vi "Save_to_Project.vi"(8 "error in (no error)":errorcluster, 9 "index in":string, 10 "buildObject":T2, 11 "IB_SoftDependency in":refnum<class "IB_SoftDependency.lvclass">) -> (0 "error out":errorcluster, 1 "index out":string, 2 "buildObject out":T2, 3 "IB_SoftDependency out":refnum<class "IB_SoftDependency.lvclass">)   [LabVIEW 2020, in "IB_SoftDependency.lvclass"]
uses:
  <vilib>/AppBuilder/IB_Classes/SoftDependency/IB_SoftDependency.lvclass
  <vilib>/AppBuilder/IB_Classes/SoftDependency/IB_SoftDependency.lvclass/IB_SoftDependency.ctl
  <vilib>/AppBuilder/IB_RW_Project/IB_RW_Project_PropBag_Action.ctl
  <resource>/Framework/Providers/API/ItemRef.ctl
  <vilib>/AppBuilder/IB_RW_Project/IB_RW_Project_SoftDep_Data.ctl
panel:
  in  "data":T1
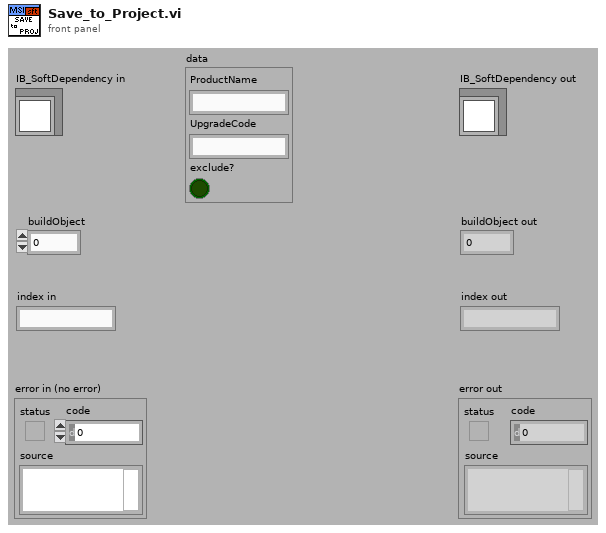
[diagram p1: front panel]
types:
  T1 = typedef "IB_RW_Project_SoftDep_Data.ctl" = cluster{"ProductName":string, "UpgradeCode":string, "exclude?":bool}
  T2 = typedef "ItemRef.ctl" = u64
  T3 = typedef "IB_RW_Project_PropBag_Action.ctl" = enum16{"read", "write", "clear", "readPrevious", "writePrevious", "clearPrevious"}
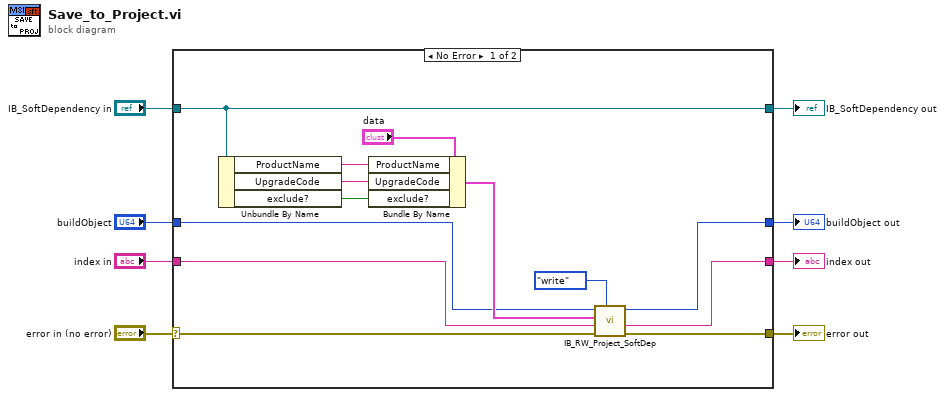
[diagram p0: block diagram]
diagram:
  n1 = case shown="No Error" "error in (no error)" {
    selector: "error in (no error)" -> [w13 w25]
    tunnel: [w12 w25] -> w7
    tunnel: [w18 w24] -> w5
    tunnel: "IB_SoftDependency in" -> [w18 w24]
    tunnel: "buildObject" -> [w17 w23]
    tunnel: [w16 w23] -> w3
    tunnel: [w15 w22] -> w2
    tunnel: "index in" -> [w14 w22]
    frame No Error {
      n2 = Unbundle By Name(w18) -> ("ProductName"=w21:string, "UpgradeCode"=w10:string, "exclude?"=w9:bool)
      n3 = Bundle By Name(cluster="data", "ProductName"=w21, "UpgradeCode"=w10, "exclude?"=w9) -> (w20:T1)
      n4 = call <vilib>:"IB_RW_Project_SoftDep.vi"("action"=IB_RW_Project_PropBag_Action."write", "error in (no error)"=w13, "index in"=w14, "dataSource in"=w20, "buildObject"=w17) -> ("error out"=w12:errorcluster, "index out"=w15:string, "buildObject out"=w16:T2)  [unwired: 4 out]
    }
    frame Error {
    }
  }
  "error out" <- w7
  "IB_SoftDependency out" <- w5
  "buildObject out" <- w3
  "index out" <- w2
